vi "Test Log Process Loop Error Message.vi"(8 "error in (no error)":errorcluster, 11 "Test Case In":refnum<class "Logger Test.lvclass">) -> (0 "error out":errorcluster, 3 "Test Case Out":refnum<class "Logger Test.lvclass">)   [LabVIEW 2021, in "Logger Test.lvclass"]
uses:
  Logger Test.lvclass
  C:/Program Files (x86)/National Instruments/LabVIEW 2021/vi.lib/Astemes/LUnit/Test Case.lvclass
  source/Framework Test Suite/Mock Log Handler/Mock Log Handler.lvclass
  C:/Git/astemes-triarc-framework/source/Framework/Logging/Logging.lvclass
  source/Framework Test Suite/Mock Process/Mock Process.lvclass
  C:/Git/astemes-triarc-framework/source/Framework/Process/Process.lvclass
  source/Framework/Process/Process.lvclass/Process.ctl
  <vilib>/Astemes/LUnit/Test Case.lvclass/Test Case.ctl
  <vilib>/Astemes/LUnit/LUnit Assertion Result.lvclass/LUnit Assertion Result.ctl
  <vilib>/Astemes/LUnit/LUnit Test Case Result.lvclass/LUnit Test Case Result.ctl
  <vilib>/Astemes/LUnit/LUnit Method Result.lvclass/LUnit Method Result.ctl
  9223215e-e84c-4064-9461-45577ae3e410.vi
  15a388cd-5dbb-4650-8421-0c4231e77477.vi
  source/Framework/Process/Public/Lifecycle/Get Lifecycle State.vi
  source/Framework/Process/Protected/Messaging/Send Message.vi
  source/Framework/Process/Private/SubVIs/Wait for finish.vi
  source/Framework/Process/Private/SubVIs/Set Lifecycle State.vi
  <vilib>/Astemes/LUnit/Palette/Pass.vi
  <vilib>/Astemes/LUnit/Palette/Fail.vi
  <vilib>/Astemes/LUnit/Compare Variants.vi
  <vilib>/Astemes/LUnit/Describe Comparison.vi
  <vilib>/Astemes/LUnit/Set Assertion Type.vi
  <vilib>/Utility/error.llb/Clear Errors.vi
  source/Framework/Process/Private/SubVIs/Handle Debug Data.vi
  <vilib>/Astemes/LUnit/Add test result.vi
  <vilib>/Astemes/LUnit/LUnit Write Passed.vi
  <vilib>/Astemes/LUnit/LUnit Write Message.vi
  <vilib>/Astemes/LUnit/LUnit Write Description.vi
  <vilib>/Astemes/LUnit/Variant to string.vi
  <vilib>/Astemes/LUnit/LUnit Write Assertion Type.vi
  source/Framework/Logging/Log Debug.vi
  <vilib>/AdvancedString/1D String Array to Delimited String.vi
  <vilib>/Utility/High Resolution Relative Seconds.vi
  <vilib>/Astemes/LUnit/LUnit Record Assertion Result.vi
  <vilib>/Astemes/LUnit/LUnit Aggregate Assertion Results.vi
  <vilib>/Astemes/LUnit/Assertion Result/LUnit Read Status.vi
  <vilib>/Astemes/LUnit/LUnit Read Message.vi
  <vilib>/Astemes/LUnit/LUnit Read Description.vi
  <vilib>/Astemes/LUnit/Method Result/LUnit Merge Status.vi
  <vilib>/Astemes/LUnit/LUnit Concatenate result strings.vi
  <vilib>/Utility/error.llb/Error Cluster From Error Code.vi
  source/Framework/Process/Public/Read Name.vi
  <vilib>/Utility/Data Type/Get Type Information.vi
  <vilib>/Utility/LVClass/Get LV Class Name.vi
  <vilib>/Astemes/LUnit/LUnit Assertion Result.lvclass
  source/Framework/Process/Process.lvclass
  Logger Test.lvclass/Logger Test.ctl
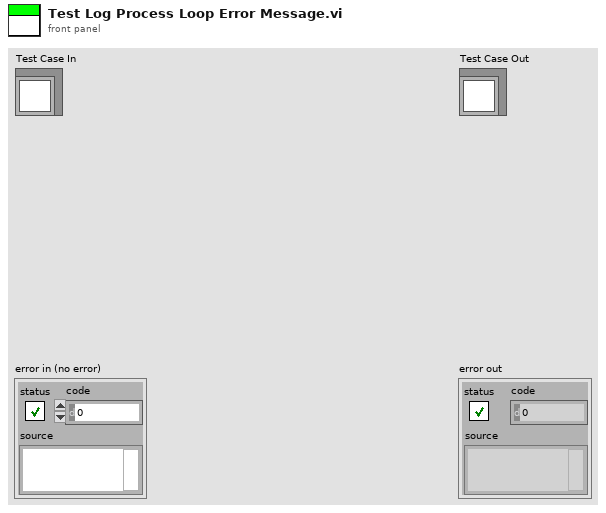
[diagram p1: front panel]
types:
  T1 = typedef "Mock Log Handler.lvclass/Log Entry.ctl" = cluster{"Level":string, "Source":string, "Message":string}
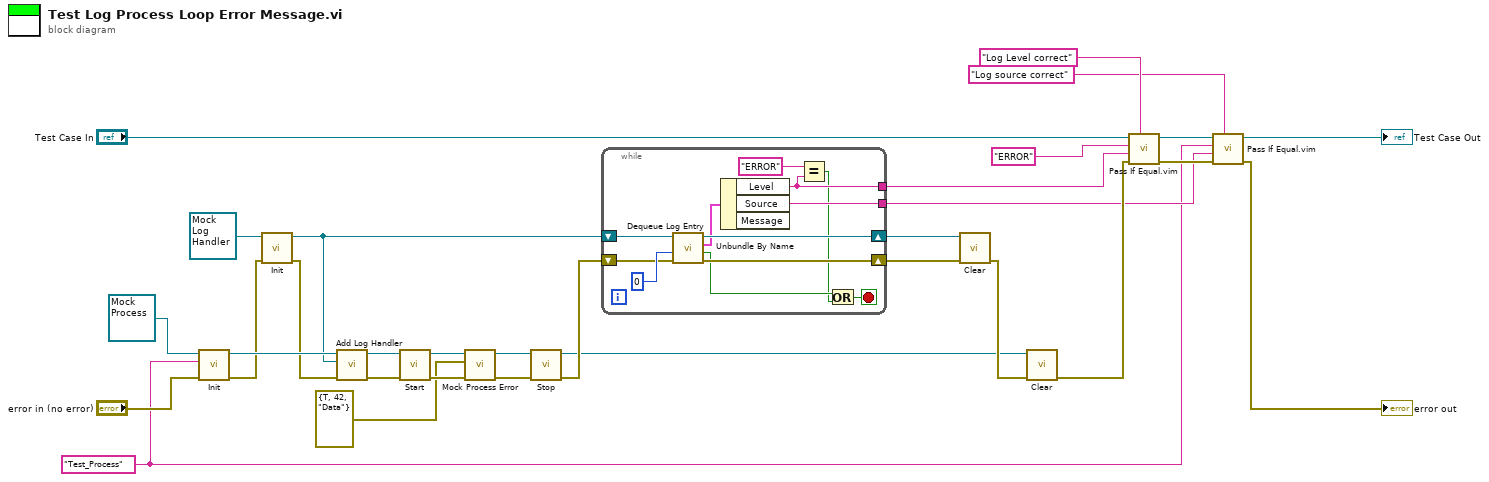
[diagram p0: block diagram]
diagram:
  w9 = "Test_Process" ("Name")
  n1 = call-dynamic "Init.vi"("error in (no error)"="error in (no error)", "Name"=w9, "Mock Process In"=refnum<class "Mock Process.lvclass"> refnum) -> ("error out"=w24:errorcluster, "Mock Process Out"=w28:refnum<class "Mock Process.lvclass">)  [unwired: 7 in]
  n2 = call-dynamic "Init.vi"("error in (no error)"=w24, "Mock Log Handler In"=refnum<class "Mock Log Handler.lvclass"> refnum ("Mock Log Handler.lvclass")) -> ("error out"=w23:errorcluster, "Mock Log Handler Out"=w20:refnum<class "Mock Log Handler.lvclass">)  [unwired: 8 in]
  n3 = call "Add Log Handler.vi"("error in (no error)"=w23, "Log Handler"=w20, "Process In"=w28) -> ("error out"=w8:errorcluster, "Process Out"=w19:refnum<class "Mock Process.lvclass">)  [unwired: 7 in]
  n4 = call "Start.vi"("error in (no error)"=w8, "Process In"=w19) -> ("error out"=w2:errorcluster, "Process Out"=w4:refnum<class "Mock Process.lvclass">)  [unwired: 7 in, 1 out]
  n5 = call "Mock Process Error.vi"("error in (no error)"=w2, "Mock Error"=errorcluster {"status"=TRUE, "code"=42, "source"="Data"} ("error in (no error)"), "Mock Process in"=w4) -> ("error out"=w5:errorcluster, "Mock Process out"=w3:refnum<class "Mock Process.lvclass">)  [unwired: 7 in]
  n6 = call "Stop.vi"("error in (no error)"=w5, "Process In"=w3) -> ("error out"=w7:errorcluster, "Process Out"=w6:refnum<class "Mock Process.lvclass">)  [unwired: 7 in, 1 out]
  n7 = while {
    tunnel: [w34] -> w17
    tunnel: [w38] -> w10
    shift-right: [w43] -> w22
    shift-left: w20 -> [w41]
    shift-right: [w42] -> w21
    shift-left: w7 -> [w37]
    stop <- w33 stop-if-true
    n8 = call "Dequeue Log Entry.vi"("error in (no error)"=w37, "timeout in ms (-1)"=0, "Mock Log Handler in"=w41) -> ("error out"=w42:errorcluster, "timed out?"=w36:bool, "Entry"=w39:T1, "Mock Log Handler out"=w43:refnum<class "Mock Log Handler.lvclass">)  [unwired: 5 in]
    n9 = Unbundle By Name(w39) -> ("Level"=w34:string, "Source"=w38:string)  [unwired: 1 out]
    n10 = Equal?(x="ERROR", y=w34) -> (x = y?=w32:bool)
    n11 = Or(x=w36, y=w32) -> (x .or. y?=w33:bool)
  }
  n12 = call-dynamic "Clear.vi"("error in (no error)"=w21, "Mock Log Handler In"=w22) -> ("error out"=w18:errorcluster)  [unwired: 9 in]
  n13 = call-dynamic "Clear.vi"("error in (no error)"=w18, "Mock Process In"=w6) -> ("error out"=w12:errorcluster)  [unwired: 9 in]
  n14 = call "Pass If Equal.vim"("Description"="Log Level correct", "error in (no error)"=w12, "Actual"=w17, "Expected"="ERROR", "LUnit Test Case In"="Test Case In") -> ("error out"=w14:errorcluster, "LUnit Test Case Out"=w30:refnum<class "Logger Test.lvclass">)  [unwired: 5 in]
  n15 = call "Pass If Equal.vim"("Description"="Log source correct", "error in (no error)"=w14, "Actual"=w10, "Expected"=w9, "LUnit Test Case In"=w30) -> ("error out"=→"error out":errorcluster, "LUnit Test Case Out"=→"Test Case Out":refnum<class "Logger Test.lvclass">)  [unwired: 5 in]
